vi "SDR Coarse Phase.vi"(5 "RMM (ohm)":dbl, 6 "MLC BLV (V)":dbl, 7 "Rmm (ohm)":dbl, 8 "error in (no error)":errorcluster, 9 "MLC WLV (V)":dbl, 10 "RM (ohm)":dbl, 11 "IVI Refnum in":refnum<k15>) -> (0 "error out":errorcluster, 2 "Numeric":dbl, 3 "IVI Refnum out":refnum<k15>)   [LabVIEW 2018]
uses:
  Globals.vi
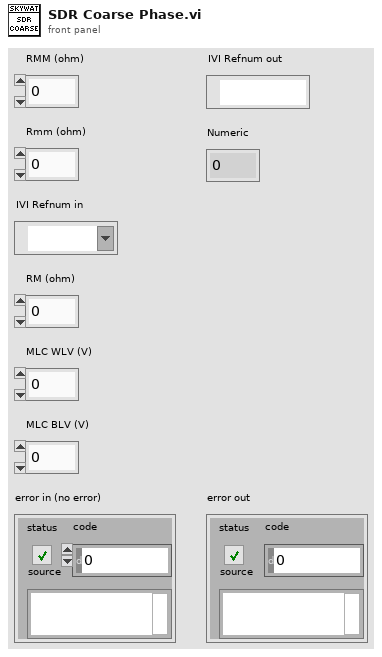
[diagram p1: front panel]
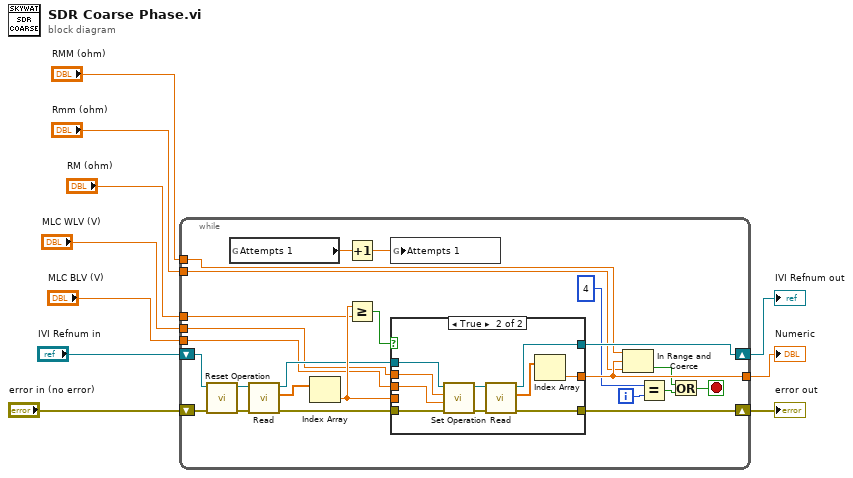
[diagram p0: block diagram]
diagram:
  n1 = while {
    tunnel: [w25] -> w3
    tunnel: "RM (ohm)" -> [w22]
    shift-right: [w23] -> w5
    shift-left: "error in (no error)" -> [w27]
    shift-right: [w24] -> w4
    shift-left: "IVI Refnum in" -> [w26]
    tunnel: "MLC WLV (V)" -> [w17]
    tunnel: "MLC BLV (V)" -> [w16]
    tunnel: "RMM (ohm)" -> [w15]
    tunnel: "Rmm (ohm)" -> [w14]
    i -> [w19]
    stop <- w21 stop-if-true
    n2 = call "Reset Operation.vi"("error in (no error)"=w27, "instrument handle"=w26) -> ("error out"=w30:errorcluster, "instrument handle out"=w28:refnum<k15>)  [unwired: 8 in]
    n3 = global read "Globals.vi" "Attempts 1"() -> (w12:dbl)
    n4 = call "Read.vi"("error in (no error)"=w30, "instrument handle"=w28) -> ("error out"=w31:errorcluster, "resistances (ohm)"=w29:dbl[], "instrument handle out"=w32:refnum<k15>)  [unwired: 6 in, 1 out]
    n5 = Index Array(array=w29) -> (element=w33:dbl)  [unwired: 1 in]
    n6 = Increment(x=w12) -> (x+1=w11:dbl)
    n7 = Greater Or Equal?(x=w33, y=w22) -> (x >= y?=w34:bool)
    n8 = global write "Globals.vi" "Attempts 1"(w11) -> ()
    n9 = case shown="True" w34 {
      tunnel: w31 -> [w37 w41]
      tunnel: [w37 w43] -> w23
      tunnel: w33 -> [w36 _]
      tunnel: [w36 w44] -> w25
      tunnel: w32 -> [w35 w47]
      tunnel: [w35 w45] -> w24
      tunnel: w17 -> [_ w39]
      tunnel: w16 -> [_ w38]
      frame False {
      }
      frame True {
        n10 = call "Set Operation.vi"("error in (no error)"=w41, "BLV"=w38, "WLV"=w39, "instrument handle"=w47) -> ("error out"=w42:errorcluster, "instrument handle out"=w46:refnum<k15>)  [unwired: 6 in]
        n11 = call "Read.vi"("error in (no error)"=w42, "instrument handle"=w46) -> ("error out"=w43:errorcluster, "resistances (ohm)"=w40:dbl[], "instrument handle out"=w45:refnum<k15>)  [unwired: 6 in, 1 out]
        n12 = Index Array(array=w40) -> (element=w44:dbl)  [unwired: 1 in]
      }
    }
    n13 = In Range and Coerce(upper limit=w15, x=w25, lower limit=w14) -> (In Range?=w13:bool)  [unwired: 1 out]
    n14 = Equal?(x=4, y=w19) -> (x = y?=w20:bool)
    n15 = Or(x=w13, y=w20) -> (x .or. y?=w21:bool)
  }
  "error out" <- w5
  "IVI Refnum out" <- w4
  "Numeric" <- w3
